vi "KeyenceCVX.Main.Scan.Trigger.vi"(8 "error in":errorcluster, 10 "TriggerNo":T4 items=["1"=1, "2"=2, "3"=3, "4"=4, "ALL"=5], 11 "Data":T1 {"Status"."TriggerNo" items=["1"=1, "2"=2, "3"=3, "4"=4, "ALL"=5]}) -> (0 "error out":errorcluster, 3 "Data out":T1 {"Status"."TriggerNo" items=["1"=1, "2"=2, "3"=3, "4"=4, "ALL"=5]})   [LabVIEW 2016]
uses:
  KeyenceCVX.Data.ctl
  KeyenceCVX.Data.Status.ctl
  KeyenceCVX.Data.Status.State.ctl
  private/controls/TriggerNo.ctl
  private/controls/RunMode.ctl
  KeyenceCVX.Data.Sets.ctl
  KeyenceCVX.CodeDetails.ctl
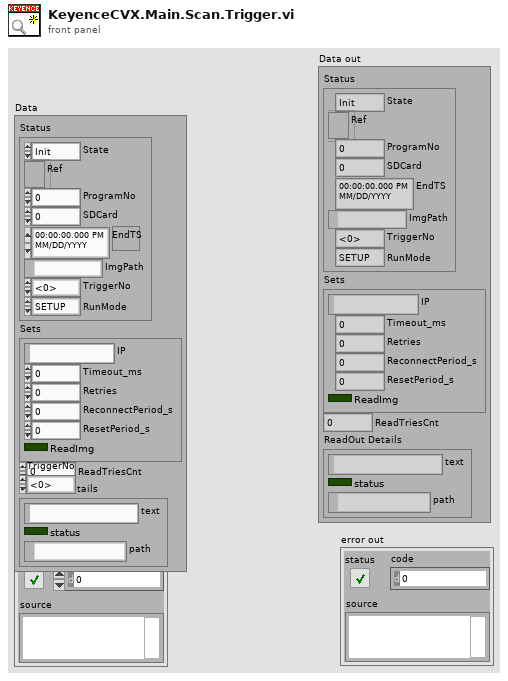
[diagram p1: front panel]
types:
  T1 = typedef "KeyenceCVX.Data.ctl" = cluster{"Status":T2, "Sets":T6, "ReadTriesCnt":u8, "ReadOut Details":T7}
  T2 = typedef "KeyenceCVX.Data.Status.ctl" = cluster{"State":T3, "Ref":refnum<k5>, "ProgramNo":u16, "SDCard":u8, "EndTS":timestamp, "ImgPath":path, "TriggerNo":T4, "RunMode":T5}
  T3 = typedef "KeyenceCVX.Data.Status.State.ctl" = enum16{"Init", "Idle", "Scan", "Reset", "ScanAck", "ChangeProgram"}
  T4 = typedef "TriggerNo.ctl" = u8
  T5 = typedef "RunMode.ctl" = enum16{"SETUP", "RUN"}
  T6 = typedef "KeyenceCVX.Data.Sets.ctl" = cluster{"IP":string, "Timeout_ms":i32, "Retries":i32, "ReconnectPeriod_s":i32, "ResetPeriod_s":i32, "ReadImg":bool}
  T7 = typedef "KeyenceCVX.CodeDetails.ctl" = cluster{"text":string, "status":bool, "path":path}
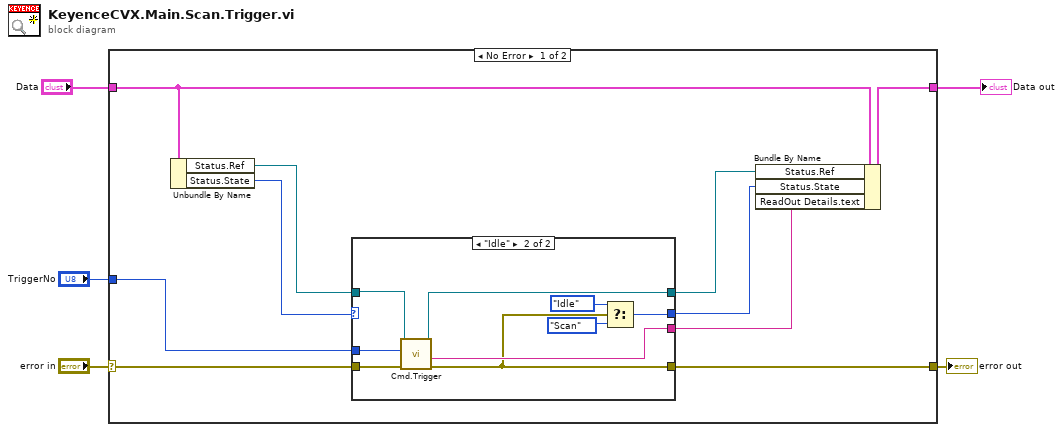
[diagram p0: block diagram]
diagram:
  n1 = case shown="No Error" "error in" {
    selector: "error in" -> [w14 w29]
    tunnel: [w8 w29] -> w4
    tunnel: "Data" -> [w11 w28]
    tunnel: [w7 w28] -> w1
    tunnel: "TriggerNo" -> [w15 _]
    frame No Error {
      n2 = Unbundle By Name(w11) -> ("Status.Ref"=w13:refnum<k5>, "Status.State"=w12:T3)
      n3 = case shown="\"Idle\"" w12 {
        selector: w12 -> [w18 _]
        tunnel: w13 -> [w17 w27]
        tunnel: w15 -> [_ w26]
        tunnel: w14 -> [w16 w25]
        tunnel: [w17 w24] -> w10
        tunnel: [w18 w19] -> w9
        tunnel: [w16 w22] -> w8
        tunnel: [_ w23] -> w6
        frame Default {
        }
        frame "Idle" {
          n4 = call "Cmd.Trigger.vi"("error in"=w25, "TriggerNo"=w26, "cID in"=w27) -> ("error out"=w22:errorcluster, "debug"=w23:string, "cID out"=w24:refnum<k5>)  [unwired: 6 in]
          n5 = Select(t=KeyenceCVX.Data.Status.State."Idle" ("Status.State"), s=w22, f=KeyenceCVX.Data.Status.State."Scan" ("Status.State")) -> (s? t:f=w19:T3)
        }
      }
      n6 = Bundle By Name(cluster=w11, "Status.Ref"=w10, "Status.State"=w9, "ReadOut Details.text"=w6) -> (w7:T1)
    }
    frame Error {
    }
  }
  "error out" <- w4
  "Data out" <- w1
